vi "templogger_server.vi"(8 "Input String":string, 11 "file (use dialog)":path) -> (0 "error out":errorcluster)   [LabVIEW 2017]
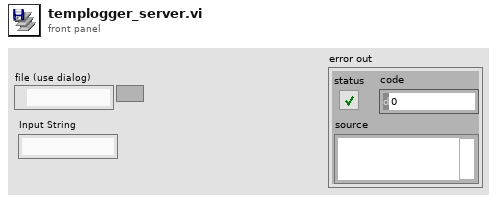
[diagram p1: front panel]
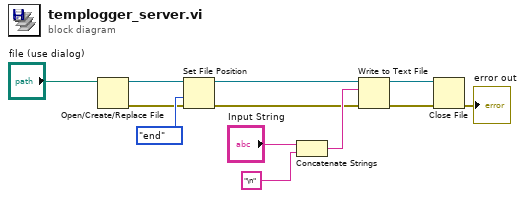
[diagram p0: block diagram]
diagram:
  n1 = Open/Create/Replace File(file path (use dialog)="file (use dialog)") -> (refnum out=w12:refnum<file>, error out=w4:errorcluster)  [unwired: 5 in, 1 out]
  n2 = Set File Position(refnum=w12, from (0:start)=enum16{"start", "end", "current"}."end", error in=w4) -> (refnum out=w10:refnum<file>, error out=w3:errorcluster)  [unwired: 1 in]
  n3 = Concatenate Strings("Input String", "\n") -> (w8:string)
  n4 = Write to Text File(file (use dialog)=w10, text=w8, error in=w3) -> (refnum out=w5:refnum<file>, error out=w2:errorcluster)  [unwired: 1 in, 1 out]
  n5 = Close File(refnum=w5, error in=w2) -> (error out=→"error out":errorcluster)  [unwired: 1 out]
